vi "CCD spectrum processing_Shaowei.vi"() -> ()   [LabVIEW 2009]
uses:
  <vilib>/Utility/file.llb/Read From Spreadsheet File (DBL).vi
panel:
  out "?":string
  out "?":string
  in  "?":bool
  out "Spectrum 2":cluster{"Y":dbl[], "Y":dbl[]}[](graph)
  in  "?":bool=TRUE
  in  "?":bool
  out "Y":sgl
  out "X":sgl
  out "MIN":dbl
  out "MAX":dbl
  out "Spectrum 1":cluster{"Y":dbl[], "Y":dbl[]}[](graph)
  in  "?":bool
  in  "?":path=path "C:/Users/S. W. Li/Desktop/0463-730.lvm"
  in  "?":path=path "C:/Users/S. W. Li/Desktop/Untitled.txt"
  in  "?":path=path "C:/Users/S. W. Li/Desktop/1.txt"
  in  "stop 2":bool
  in  "?":bool
  in  "stop":bool
  out "?":ext=1340.0
  in  "to":dbl=950.0
  in  "From":dbl=550.0
  in  "?":bool
  in  "?":i32(ring)=1 items=["nm"=1, "eV"=2, "cm-1"=3, "Pixel #"=4]
  # "Input File"
  # "2 Files"
  # "1 File"
  # "1st"
  # "2nd"
  # "Active Window"
  # "#1"
  # "#2"
  # "Spectra Range"
  # "nm"
  # "nm"
  # "# of Pixel"
  # "X unit"
  # "Cosmic Ray Removal"
  # "NO"
  # "YES"
  # "Value"
  # "Position"
  # "Save File"
  # "NO"
  # "YES"
  # "Descending"
  # "Sort Data by X"
  # "File Name"
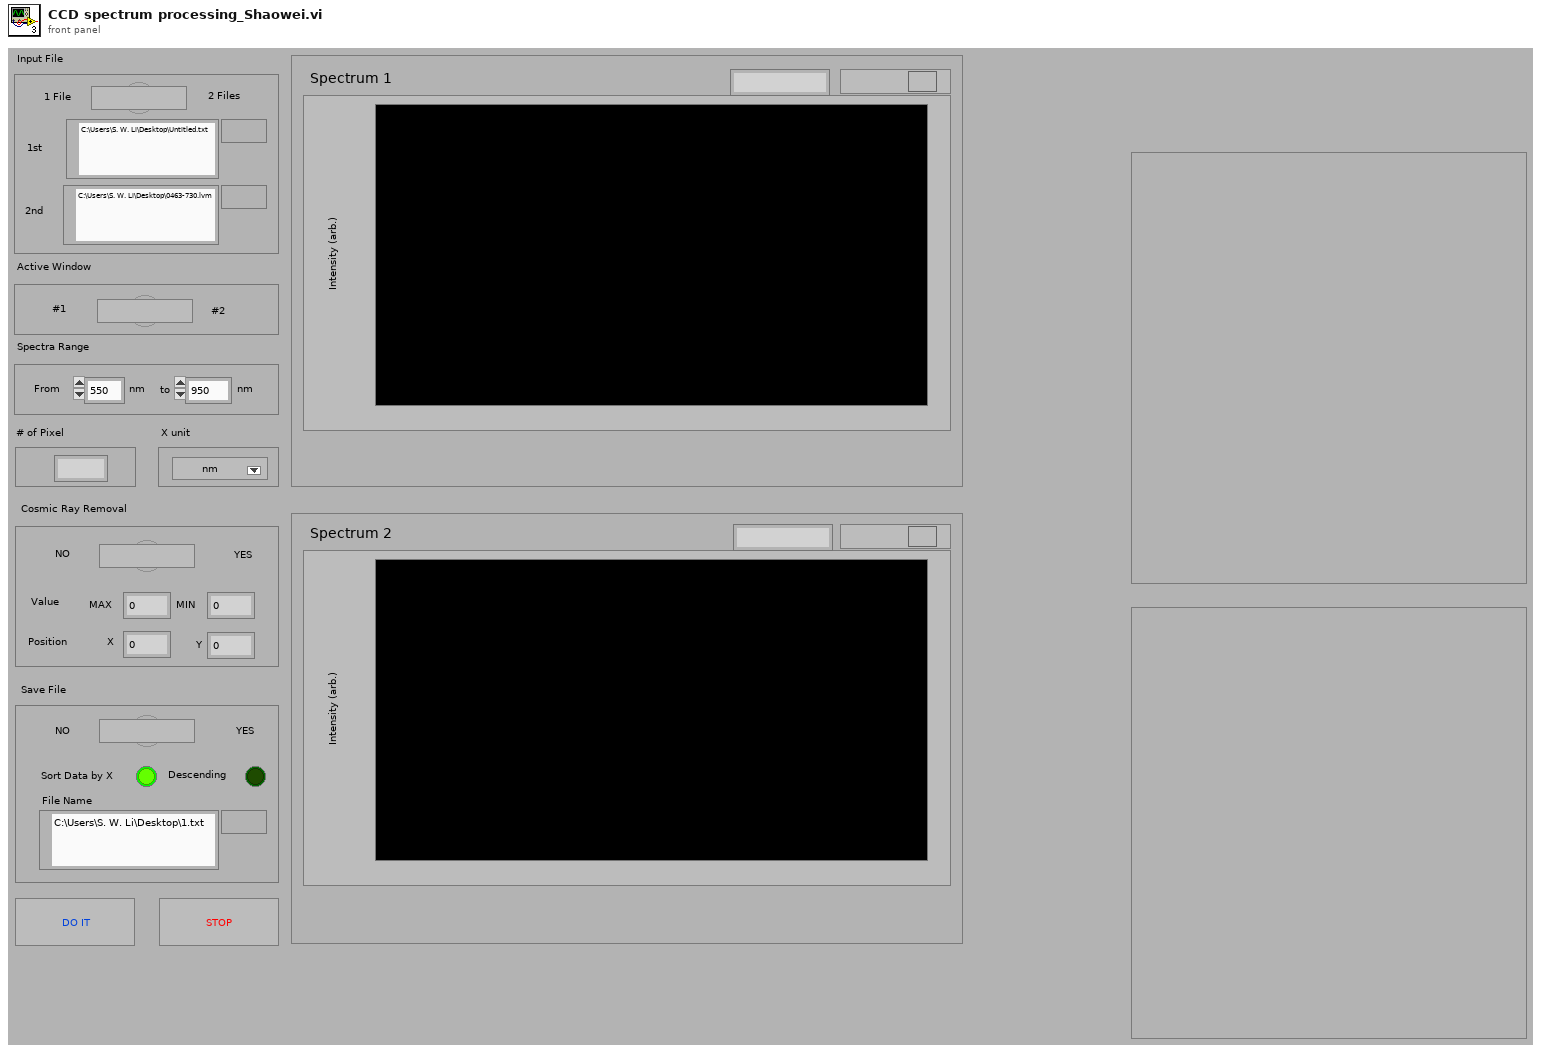
[diagram p1: front panel]
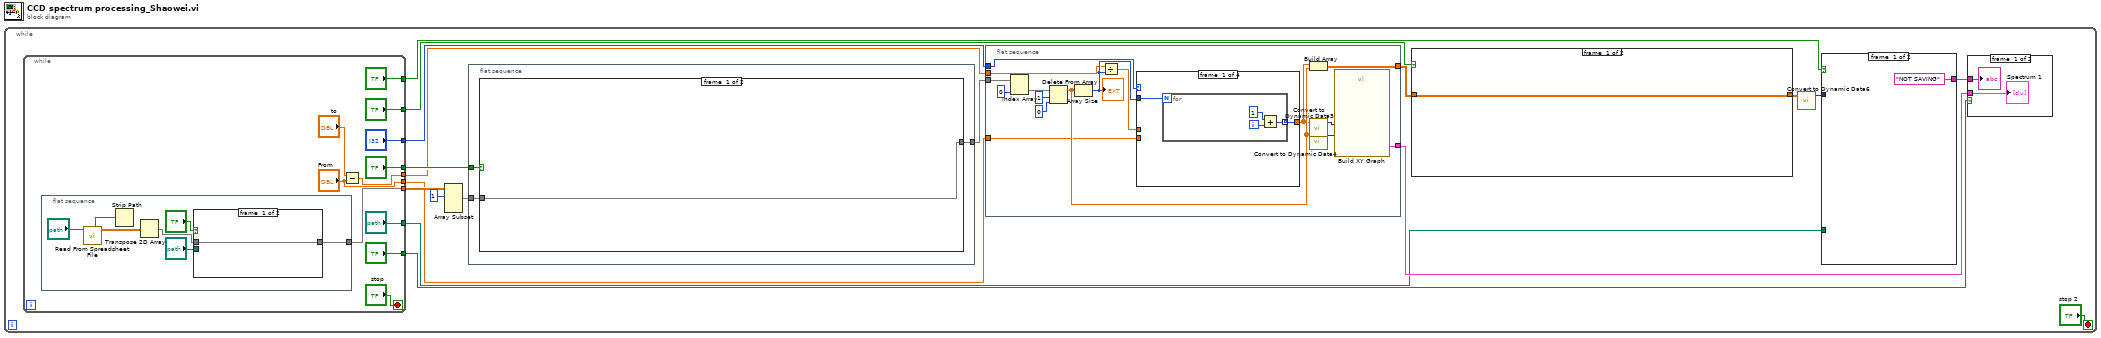
[diagram p0: block diagram]
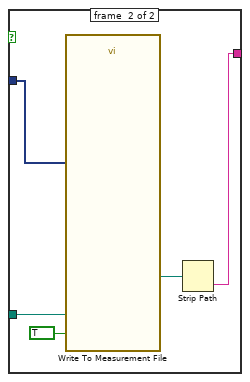
[diagram p2: hidden frame]
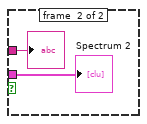
[diagram p3: hidden frame]
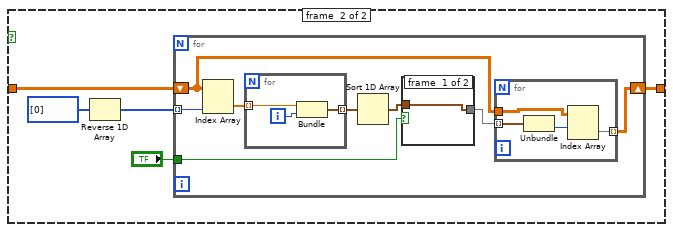
[diagram p4: hidden frame]
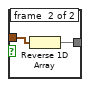
[diagram p5: hidden frame]
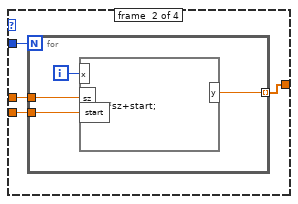
[diagram p6: hidden frame]
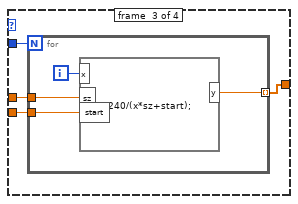
[diagram p7: hidden frame]
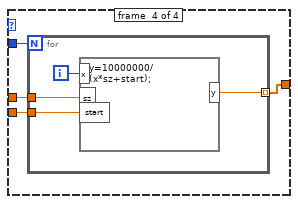
[diagram p8: hidden frame]
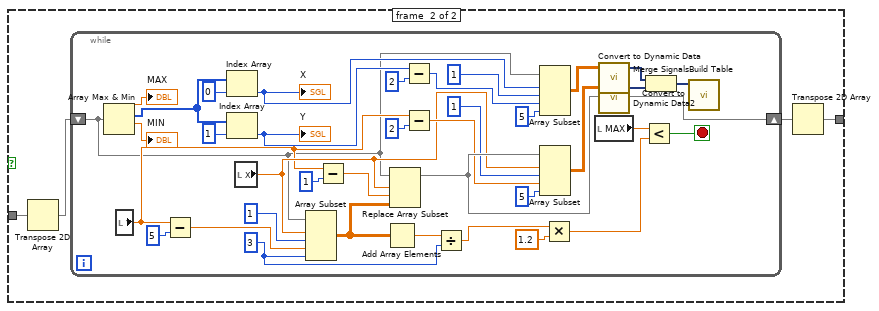
[diagram p9: hidden frame]
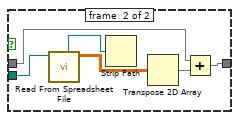
[diagram p10: hidden frame]
diagram:
  n1 = while {
    stop <- "stop 2" stop-if-true
    n2 = while {
      tunnel: ["?"] -> w2
      tunnel: ["?"] -> w16
      tunnel: [w151] -> w11
      tunnel: ["From"] -> w10
      tunnel: ["?"] -> w3
      tunnel: [w146] -> w14
      tunnel: ["?"] -> w12
      tunnel: ["?"] -> w7
      tunnel: ["?"] -> w4
      stop <- "stop" stop-if-true
      n3 = flat-sequence {
        tunnel: [w157] -> w146
        frame #0 {
          n4 = call-poly <vilib>:"Read From Spreadsheet File.vi"("file path (dialog if empty)"="?") -> ("all rows"=w160:dbl[][], "new file path (Not A Path if cancelled)"=w159:path)  [unwired: 6 in, 3 out]
          n5 = Strip Path(path=w159) -> ()  [unwired: 2 out]
          n6 = Transpose 2D Array(2D array=w160) -> (transposed array=w158:dbl[][])
          n7 = case shown="False" "?" {
            tunnel: w158 -> [w161 w166]
            tunnel: [w161 w165] -> w157
            tunnel: "?" -> [_ w162]
            frame #0 {
            }
            frame #1 {
              n8 = call-poly <vilib>:"Read From Spreadsheet File.vi"("file path (dialog if empty)"=w162) -> ("all rows"=w164:dbl[][], "new file path (Not A Path if cancelled)"=w167:path)  [unwired: 6 in, 3 out]
              n9 = Strip Path(path=w167) -> ()  [unwired: 2 out]
              n10 = Transpose 2D Array(2D array=w164) -> (transposed array=w163:dbl[][])
              n11 = Add(x=w166, y=w163) -> (x+y=w165:dbl[][])
            }
          }
        }
      }
      n12 = Subtract(x="to", y="From") -> (x-y=w151:dbl)
    }
    n13 = Array Subset(array=w14, index (row)=1) -> (w18:dbl[][])  [unwired: 3 in]
    n14 = flat-sequence {
      tunnel: w18 -> [w100]
      tunnel: w16 -> [w99]
      tunnel: [w98] -> w13
      frame #0 {
        n15 = case shown="True" w99 {
          tunnel: w100 -> [w101 w105]
          tunnel: [w101 w103] -> w98
          frame #0 {
          }
          frame #1 {
            n16 = Transpose 2D Array(2D array=w105) -> (transposed array=w104:dbl[][])
            n17 = while {
              shift-right: [w142] -> w102
              shift-left: w104 -> [w106]
              stop <- w121 stop-if-true
              w119 = 3
              n18 = Array Max & Min(array=w106) -> (max value=→"MAX":dbl, max index (indices)=w140:i32[], min value=→"MIN":dbl)  [unwired: 1 out]
              n19 = local read "Y"() -> (w108:sgl)
              n20 = Subtract(x=w108, y=5) -> (x-y=w136:sgl)
              n21 = Index Array(array=w140, index=0) -> (element=w113:i32)
              "X" <- w113
              n22 = Index Array(array=w140, index=1) -> (element=w112:i32)
              "Y" <- w112
              n23 = local read "X"() -> (w109:sgl)
              n24 = Array Subset(array=w106, index (row)=w109, length (row)=1, index (col)=w136, length (col)=w119) -> (w118:dbl[][])
              n25 = Subtract(x=w108, y=1) -> (x-y=w135:sgl)
              n26 = Add Array Elements(numeric array=w118) -> (sum=w120:dbl)
              n27 = Replace Array Subset(array=w106, new element=w118, index (row)=w109, index (col)=w135) -> (w142:dbl[][])
              n28 = Subtract(x=w112, y=2) -> (x-y=w126:i32)
              n29 = Subtract(x=w108, y=2) -> (x-y=w131:sgl)
              n30 = Divide(x=w120, y=w119) -> (x/y=w117:dbl)
              n31 = Array Subset(array=w106, index (row)=w113, length (row)=1, index (col)=w126, length (col)=5) -> (w124:dbl[][])
              n32 = Array Subset(array=w142, index (row)=w109, length (row)=1, index (col)=w131, length (col)=5) -> (w129:dbl[][])
              n33 = Multiply(x=w117, y=1.2) -> (x*y=w122:dbl)
              n34 = local read "MAX"() -> (w107:dbl)
              n35 = call "Convert to Dynamic Data"("2D Array"=w124) -> ("Dynamic Data Type"=w116:dynamicdata)  [unwired: 3 in]
              n36 = call "Convert to Dynamic Data2"("2D Array"=w129) -> ("Dynamic Data Type"=w114:dynamicdata)  [unwired: 3 in]
              n37 = Less?(x=w107, y=w122) -> (x < y?=w121:bool)
              n38 = Merge Signals(w116, w114) -> (w115:dynamicdata)
              n39 = call "Build Table"("Signals"=w115) -> ()  [unwired: 9 in, 2 out]
            }
            n40 = Transpose 2D Array(2D array=w102) -> (transposed array=w103:dbl[][])
          }
        }
      }
    }
    n41 = flat-sequence {
      tunnel: w13 -> [w68]
      tunnel: [w60] -> w9
      tunnel: w12 -> [w58]
      tunnel: w11 -> [w56]
      tunnel: w10 -> [w55]
      tunnel: [w53] -> w5
      frame #0 {
        n42 = Index Array(array=w68, index (col)=0) -> (element=w63:dbl[])  [unwired: 1 in]
        n43 = Delete From Array(array=w63, length=1, index=0) -> (array with subset deleted=w62:dbl[])  [unwired: 1 out]
        n44 = Array Size(array=w62) -> (size(s)=w57:i32)
        "?" <- w57
        n45 = Divide(x=w56, y=w57) -> (x/y=w54:dbl)
        n46 = case shown="4, Default" w58 {
          tunnel: w57 -> [w70 w77 w85 w93]
          tunnel: [w69 w76 w84 w92] -> w61
          tunnel: w55 -> [_ w75 w83 w91]
          tunnel: w54 -> [_ w74 w82 w90]
          frame #0 {
            n47 = for {
              N: w70 -> [_]
              tunnel: [w71] -> w69 mode=indexing
              i -> [w72]
              n48 = Add(x=1, y=w72) -> (x+y=w71:i32)
            }
          }
          frame #1 {
            n49 = for {
              N: w77 -> [_]
              tunnel: [w78] -> w76 mode=indexing
              tunnel: w75 -> [w80]
              tunnel: w74 -> [w79]
              i -> [w81]
              n50 = formula code="y=x*sz+start;"("x"=w81, "sz"=w79, "start"=w80) -> ("y"=w78:dbl)
            }
          }
          frame #2 {
            n51 = for {
              N: w85 -> [_]
              tunnel: [w86] -> w84 mode=indexing
              tunnel: w83 -> [w88]
              tunnel: w82 -> [w87]
              i -> [w89]
              n52 = formula code="y=1240/(x*sz+start);"("x"=w89, "sz"=w87, "start"=w88) -> ("y"=w86:dbl)
            }
          }
          frame #3 {
            n53 = for {
              N: w93 -> [_]
              tunnel: [w94] -> w92 mode=indexing
              tunnel: w91 -> [w96]
              tunnel: w90 -> [w95]
              i -> [w97]
              n54 = formula code="y=10000000/(x*sz+start);"("x"=w97, "sz"=w95, "start"=w96) -> ("y"=w94:dbl)
            }
          }
        }
        n55 = Build Array(w61, w62) -> (w60:dbl[][])
        n56 = call "Convert to Dynamic Data3"("Array"=w61) -> ("Dynamic Data Type"=w67:dynamicdata)  [unwired: 3 in]
        n57 = call "Convert to Dynamic Data4"("Array"=w62) -> ("Dynamic Data Type"=w66:dynamicdata)  [unwired: 3 in]
        n58 = call "Build XY Graph"("Y Input"=w66, "X Input"=w67) -> ("XY Graph"=w53:cluster{"Y":dbl[], "Y":dbl[]}[])  [unwired: 8 in, 1 out]
      }
    }
    n59 = case shown="True" w7 {
      tunnel: w9 -> [w29 w31]
      tunnel: [w29 w30] -> w6
      frame #0 {
      }
      frame #1 {
        n60 = Reverse 1D Array(array=i32[] [0] ("Priority Columns (0)")) -> (reversed array=w33:i32[])
        n61 = for {
          shift-right: [w36] -> w30
          shift-left: w31 -> [w38]
          tunnel: w33 -> [w35] mode=indexing
          tunnel: "?" -> [w37]
          n62 = Index Array(array=w38, index (col)=w35) -> (element=w40:dbl[])  [unwired: 1 in]
          n63 = for {
            tunnel: w40 -> [w50] mode=indexing
            tunnel: [w52] -> w39 mode=indexing
            i -> [w51]
            n64 = Bundle("y"=w50, w51) -> (w52:cluster{"y":dbl, i32})  [unwired: 1 out]
          }
          n65 = Sort 1D Array(array=w39) -> (sorted array=w42:cluster{"y":dbl, i32}[])
          n66 = case shown="True" w37 {
            tunnel: [w43 w44] -> w41
            tunnel: w42 -> [w43 w45]
            frame #0 {
            }
            frame #1 {
              n67 = Reverse 1D Array(array=w45) -> (reversed array=w44:cluster{"y":dbl, i32}[])
            }
          }
          n68 = for {
            tunnel: w41 -> [w49] mode=indexing
            tunnel: w38 -> [w48]
            tunnel: [w46] -> w36 mode=indexing
            n69 = Unbundle(w49) -> (w47:i32)  [unwired: 1 out]
            n70 = Index Array(array=w48, index (row)=w47) -> (element=w46:dbl[])  [unwired: 1 in]
          }
        }
      }
    }
    n71 = call "Convert to Dynamic Data6"("2D Array"=w6) -> ("Dynamic Data Type"=w8:dynamicdata)  [unwired: 3 in]
    n72 = case shown="True" w3 {
      tunnel: w8 -> [_ w24]
      tunnel: w2 -> [_ w23]
      tunnel: ["NOT SAVING" ("name") w20] -> w1
      frame #0 {
      }
      frame #1 {
        n73 = call "Write To Measurement File"("Signals"=w24, "Reset"=TRUE, "Filename"=w23) -> ("Filename Out"=w21:path)  [unwired: 14 in, 2 out]
        n74 = Strip Path(path=w21) -> (name=w20:string)  [unwired: 1 out]
      }
    }
    n75 = case shown="False" w4 {
      tunnel: w5 -> [w26 w28]
      tunnel: w1 -> [w25 w27]
      frame #0 {
        "Spectrum 1" <- w26
        "?" <- w25
      }
      frame #1 {
        "Spectrum 2" <- w28
        "?" <- w27
      }
    }
  }
